vi "GOOP_VirtualFolder_Item_OnCommand.vi"(10 "Command Tag":string, 11 "Object":u64) -> ()   [LabVIEW 2020]
uses:
  ClassProviders/Provider_BaseClassInterface/ClassWriter_class/ClassWriter.lvclass
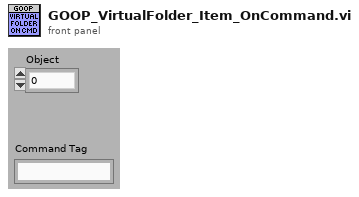
[diagram p1: front panel]
types:
  T1 = enum8{"No dynamic dispatch VIs", "Include nearest implementation", "Include all overrides"}
  T2 = typedef "GDSIconEditor_FileNameFilter.ctl" = cluster{"String/Match Pattern to remove":string[], "Strings To Convert From - To":cluster{"From":string, "To":string}[]}
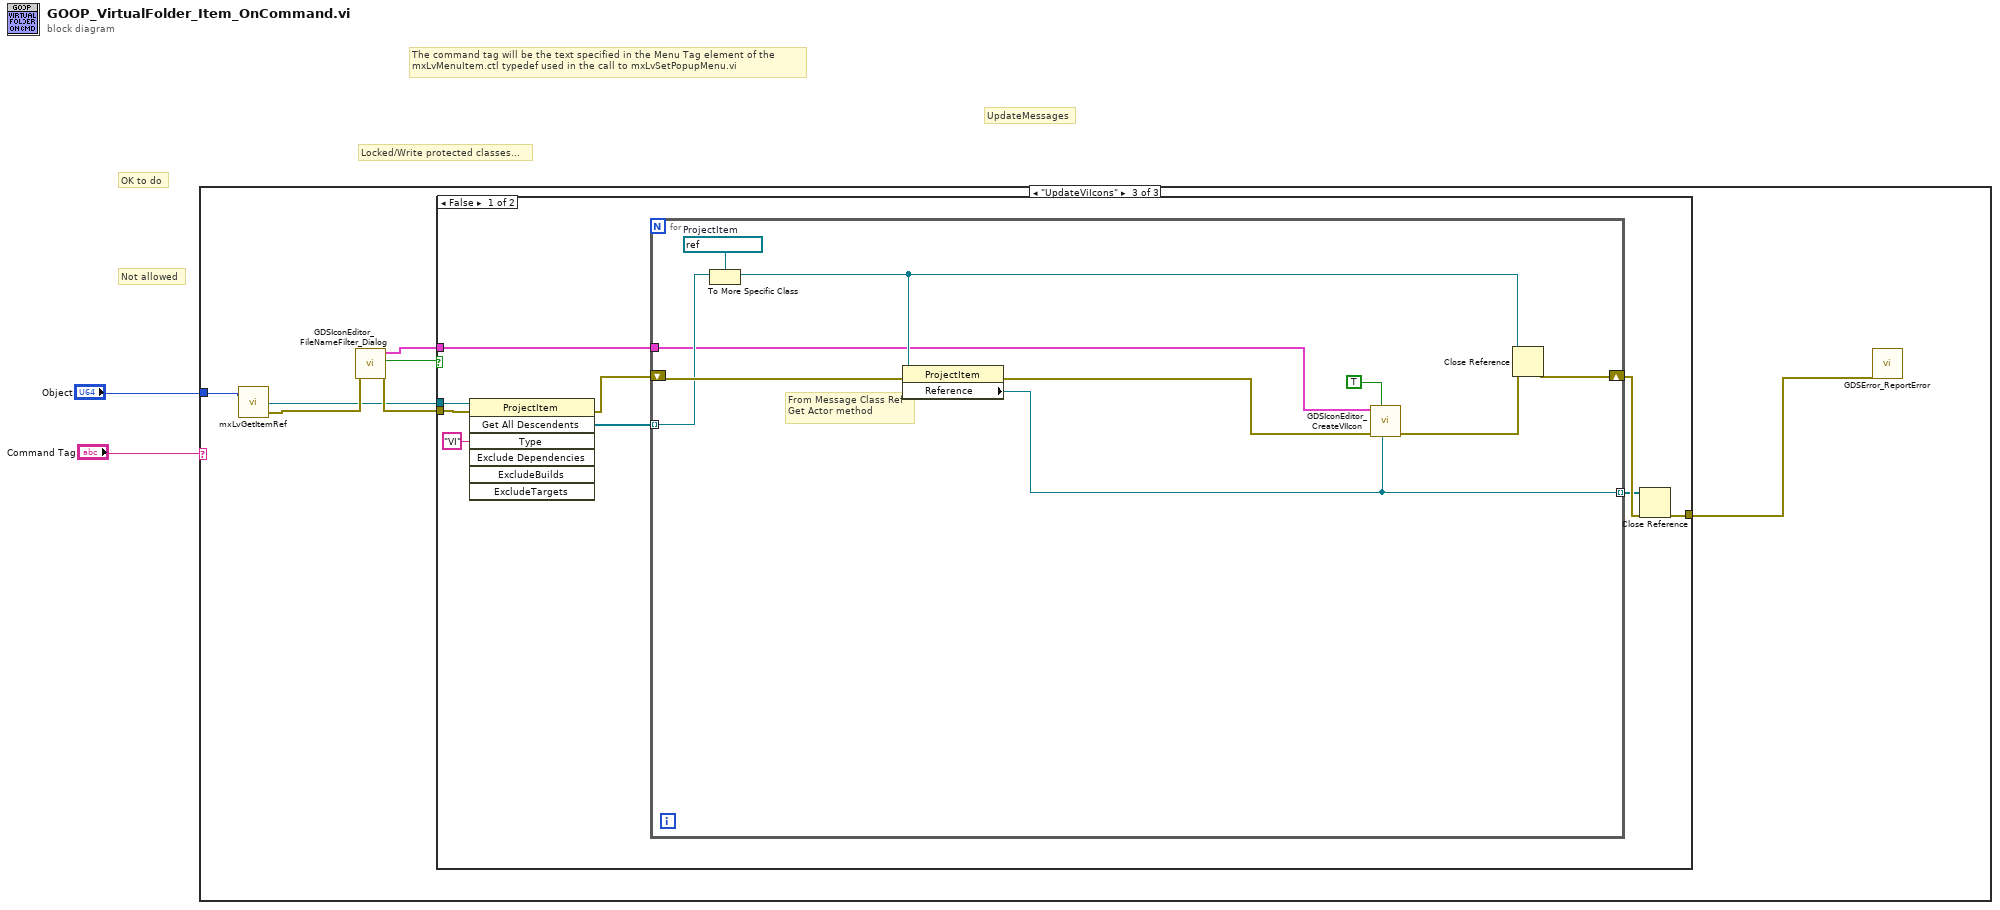
[diagram p0: block diagram]
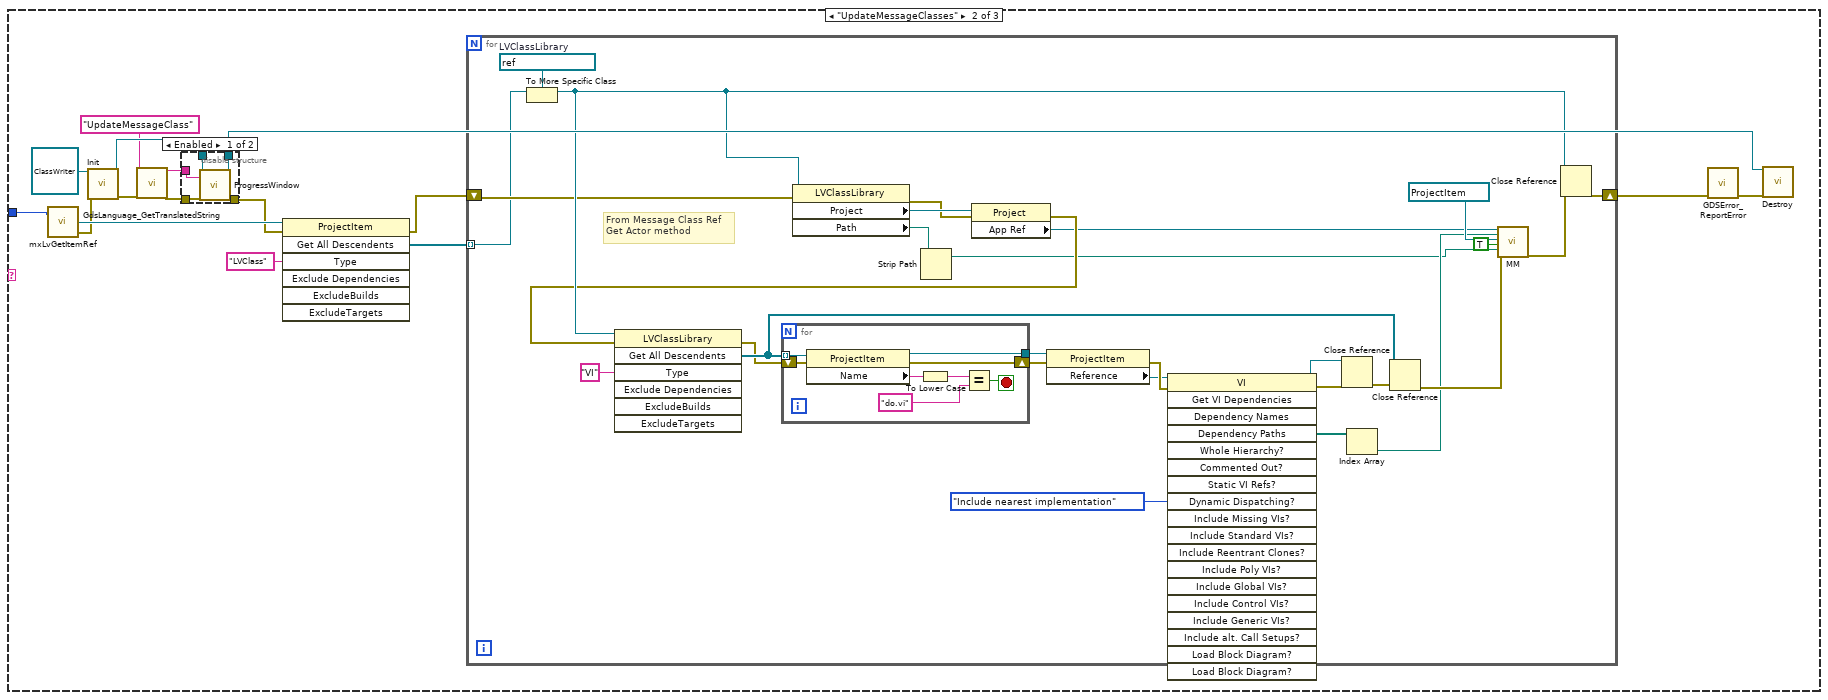
[diagram p3: hidden frame]
diagram:
  # "UpdateMessages"
  # "Not allowed"
  # "OK to do"
  # "Locked/Write protected classes..."
  # "The command tag will be the text specified in the Menu Tag element of the \nmxLvMenuItem.ctl typedef used in the call to mxLvSetPopupMenu.vi"
  n1 = case shown="\"UpdateViIcons\"" "Command Tag" {
    tunnel: "Object" -> [_ w18 w68]
    frame Default {
    }
    frame "UpdateMessageClasses" {
      n2 = call <resource>:"mxLvGetItemRef.vi"("Item"=w18) -> ("Item Refnum"=w17:refnum<vi>, "error out"=w6:errorcluster)  [unwired: 1 in, 1 out]
      n3 = call-dynamic "Init.vi"("ClassWriter in"=refnum<class "ClassWriter.lvclass"> refnum, "error in (no error)"=w6) -> ("ClassWriter out"=w14:refnum<class "ClassWriter.lvclass">, "error out"=w11:errorcluster)  [unwired: 16 in]
      n4 = call "GdsLanguage_GetTranslatedString.vi"("StringID(s)"="UpdateMessageClass" ("Message(Exit)"), "error in (no error)"=w11) -> ("FirstStringOut"=w10:string, "error out"=w12:errorcluster)  [unwired: 14 in, 2 out]
      n5 = disable-structure shown="Enabled" {
        disable-tunnel: w10 -> [w59 _]
        disable-tunnel: [w58 w61] -> w4
        disable-tunnel: w12 -> [w57 w61]
        disable-tunnel: w14 -> [w56 w60]
        disable-tunnel: [w55 w60] -> w15
        frame Enabled {
          n6 = call-dynamic "ProgressWindow.vi"("ClassWriter in"=w56, "Message(Exit)"=w59, "error in (no error)"=w57) -> ("ClassWriter out"=w55:refnum<class "ClassWriter.lvclass">, "error out"=w58:errorcluster)  [unwired: 15 in]
        }
        frame Disabled {
        }
      }
      n7 = invoke class="ProjectItem" method="Get All Descendents"(reference=w17, error in=w4, "Type"="LVClass") -> (error out=w5:errorcluster, "All Descendents"=w7:refnum<vi>[])  [unwired: 4 in, 5 out]
      n8 = for {
        tunnel: w7 -> [w19] mode=indexing
        shift-right: [w21] -> w8
        shift-left: w5 -> [w44]
        w20 = refnum<vi> refnum  # LVClassLibrary
        # "From Message Class Ref\nGet Actor method"
        n9 = To More Specific Class(target class=w20, reference=w19) -> (specific class reference=w45:refnum<vi>)  [unwired: 1 in, 1 out]
        n10 = property class="LVClassLibrary"(reference=w45, error in=w44) -> (error out=w22:errorcluster, "Project"=w23:refnum<vi>, "Path"=w26:path)  [unwired: 1 out]
        n11 = Strip Path(path=w26) -> (stripped path=w27:path)  [unwired: 1 out]
        n12 = property class="Project"(reference=w23, error in=w22) -> (error out=w33:errorcluster, "App Ref"=w24:refnum<vi>)  [unwired: 1 out]
        n13 = invoke class="LVClassLibrary" method="Get All Descendents"(reference=w45, error in=w33, "Type"="VI") -> (error out=w31:errorcluster, "All Descendents"=w39:refnum<vi>[])  [unwired: 4 in, 5 out]
        n14 = for {
          tunnel: w39 -> [w54] mode=indexing
          tunnel: [w50] -> w29
          shift-right: [w49] -> w30
          shift-left: w31 -> [w48]
          stop <- w47 stop-if-true
          n15 = property class="ProjectItem"(reference=w54, error in=w48) -> (reference out=w50:refnum<vi>, error out=w49:errorcluster, "Name"=w53:string)
          n16 = To Lower Case(string=w53) -> (all lower case string=w52:string)
          n17 = Equal?(x=w52, y="do.vi") -> (x = y?=w47:bool)
        }
        n18 = property class="ProjectItem"(reference=w29, error in=w30) -> (error out=w35:errorcluster, "Reference"=w32:refnum<vi>)  [unwired: 1 out]
        n19 = invoke class="VI" method="Get VI Dependencies"(reference=w32, error in=w35, "Dynamic Dispatching?"=T1."Include nearest implementation") -> (reference out=w37:refnum<vi>, error out=w36:errorcluster, "Dependency Paths"=w40:path[])  [unwired: 16 in, 16 out]
        n20 = Close Reference(reference=w37, error in (no error)=w36) -> (error out=w38:errorcluster)
        n21 = Index Array(array=w40) -> (element=w41:path)  [unwired: 1 in]
        n22 = Close Reference(reference=w39, error in (no error)=w38) -> (error out=w42:errorcluster)
        n23 = call "MM.vi"("AppInst"=w24, "ActorMethod"=w41, "ActorClassItemRef(Don't Delete)"=refnum<vi> refnum, "OnlyUpdate(if needed,False)"=TRUE ("OnlyUpdate(if needed)"), "Destination Path"=w27, "error in"=w42) -> ("error out"=w43:errorcluster)  [unwired: 13 in]
        n24 = Close Reference(reference=w45, error in (no error)=w43) -> (error out=w21:errorcluster)
      }
      n25 = call "GDSError_ReportError.vi"("error in (no error)"=w8) -> ("error out"=w13:errorcluster)  [unwired: 18 in]
      n26 = call-dynamic "Destroy.vi"("ClassWriter.lvclass"=w15, "error in (no error)"=w13) -> ()  [unwired: 17 in, 1 out]
    }
    frame "UpdateViIcons" {
      n27 = call <resource>:"mxLvGetItemRef.vi"("Item"=w68) -> ("Item Refnum"=w65:refnum<vi>, "error out"=w67:errorcluster)  [unwired: 1 in, 1 out]
      n28 = call "GDSIconEditor_FileNameFilter_Dialog.vi"("error in"=w67) -> ("error out"=w66:errorcluster, "Cancelled"=w64:bool, "FileNameConverions"=w62:T2)  [unwired: 8 in]
      n29 = case shown="False" w64 {
        tunnel: w66 -> [w74 w88]
        tunnel: w65 -> [w73 _]
        tunnel: [w70 w88] -> w63
        tunnel: w62 -> [w69 _]
        frame False {
          n30 = invoke class="ProjectItem" method="Get All Descendents"(reference=w73, error in=w74, "Type"="VI") -> (error out=w75:errorcluster, "All Descendents"=w76:refnum<vi>[])  [unwired: 4 in, 5 out]
          n31 = for {
            tunnel: w76 -> [w83] mode=indexing
            shift-right: [w85] -> w72
            shift-left: w75 -> [w86]
            tunnel: [w80] -> w71 mode=indexing
            tunnel: w69 -> [w78]
            w84 = refnum<vi> refnum  # ProjectItem
            # "From Message Class Ref\nGet Actor method"
            n32 = To More Specific Class(target class=w84, reference=w83) -> (specific class reference=w87:refnum<vi>)  [unwired: 1 in, 1 out]
            n33 = property class="ProjectItem"(reference=w87, error in=w86) -> (error out=w79:errorcluster, "Reference"=w80:refnum<vi>)  [unwired: 1 out]
            n34 = call "GDSIconEditor_CreateVIIcon.vi"("ViRef(IgnoreIfNotWired)"=w80, "AutomaticUpdateNoQuestionsAsked(False)"=TRUE, "error in (no error)"=w79, "FileNameConverions"=w78) -> ("error out"=w81:errorcluster)  [unwired: 7 in]
            n35 = Close Reference(reference=w87, error in (no error)=w81) -> (error out=w85:errorcluster)
          }
          n36 = Close Reference(reference=w71, error in (no error)=w72) -> (error out=w70:errorcluster)
        }
        frame True {
        }
      }
      n37 = call "GDSError_ReportError.vi"("error in (no error)"=w63) -> ()  [unwired: 18 in, 1 out]
    }
  }
